vi "Read keys.vi"(8 "error in (no error)":errorcluster, 11 "Parameter to Hardware Map in":refnum<class "Parameter to Hardware Map.lvclass">) -> (0 "error out":errorcluster, 2 "Keys":string[](array[string]), 3 "Parameter to Hardware Map out":refnum<class "Parameter to Hardware Map.lvclass">)   [LabVIEW 2020, in "RxnRover.lvlib" / "Parameter to Hardware Map.lvclass"]
doc: "Returns the underlying unordered_map array."
uses:
  Parameter to Hardware Map.lvclass
  Parameter to Hardware Map.lvclass/Parameter to Hardware Map.ctl
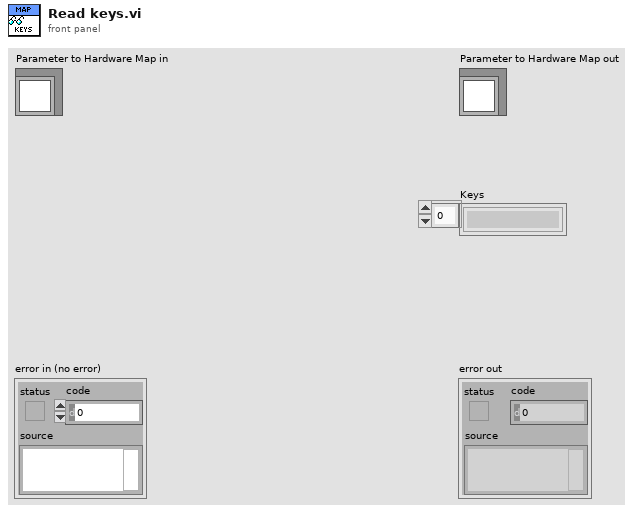
[diagram p1: front panel]
types:
  T1 = typedef "RxnRover.lvlib/Parameter to Hardware Map.lvclass/Pair.ctl" = cluster{"key":string, "values":refnum<class "Generic Plugin.lvclass">[]}
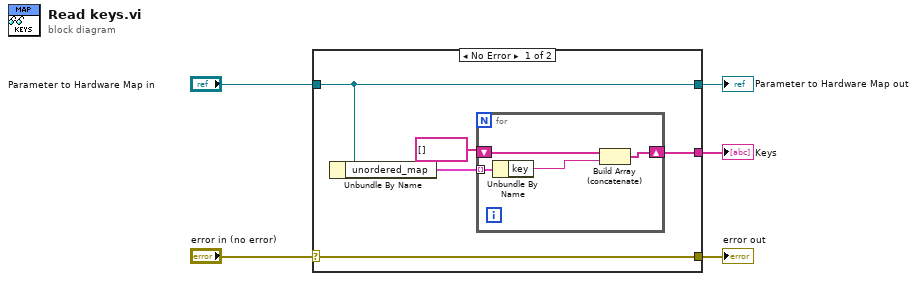
[diagram p0: block diagram]
diagram:
  n1 = case shown="No Error" "error in (no error)" {
    selector: "error in (no error)" -> [w10 w15]
    tunnel: [w10 w15] -> w4
    tunnel: [w9 w16] -> w2
    tunnel: "Parameter to Hardware Map in" -> [w9 w16]
    tunnel: [w7 _] -> w1
    frame No Error {
      n2 = Unbundle By Name(w9) -> ("unordered_map"=w8:T1[])
      n3 = for {
        tunnel: w8 -> [w14] mode=indexing
        shift-right: [w11] -> w7
        shift-left: string[] [] -> [w12]
        n4 = Unbundle By Name(w14) -> ("key"=w13:string)
        n5 = Build Array (concatenate)(w12, w13) -> (w11:string[])
      }
    }
    frame Error {
    }
  }
  "error out" <- w4
  "Parameter to Hardware Map out" <- w2
  "Keys" <- w1
